vi "WireSelectionControl.vi"() -> ()   [LabVIEW 2020]
uses:
  resource/Framework/Providers/Open_GDS/SubVIs/GOOP_WireConfigurationType.ctl
  resource/Framework/Providers/Open_GDS/SubVIs/GOOP_WirePattern.ctl
  <vilib>/numeric/Random Number (Range) U64.vi
  <vilib>/numeric/sub_Random U32.vi
panel:
  out "Array":T1(array[cluster])
  out "Picture":picture
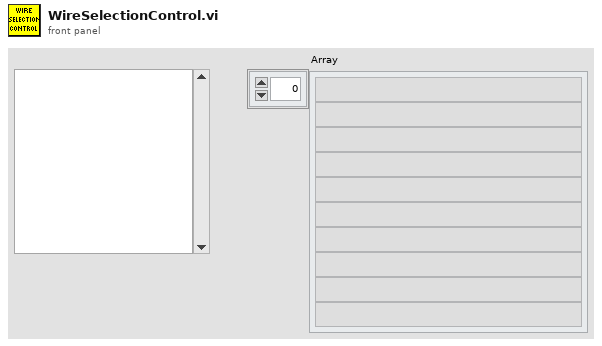
[diagram p1: front panel]
types:
  T1 = cluster{"Name":string, "Wire":picture, "Bg":picture}[]
  T2 = cluster{"left":i16, "top":i16, "right":i16, "bottom":i16}
  T3 = typedef "GOOP_WireConfigurationType.ctl" = cluster{"Edge thickness":i32, "Edge color":u32, "Center thickness":i32, "Center pattern":T4, "CenterColor1":u32, "CenterColor2":u32, "Tunnels and terminals colors":u32}
  T4 = typedef "GOOP_WirePattern.ctl" = enum16{"Solid", "Large dash", "Small dash"}
  T5 = cluster{"Width":i16, "Style":enum32{"Solid", "Dash", "Dot", "DashDot", "DashDotDot"}}
  T6 = cluster{"ImageEnd-Y":i32, i32, "rect":cluster{"left":i16, "top":i16, "right":i16, "bottom":i16}}
  T7 = cluster{string, "WirePictureOut":picture, "new picture":picture}
  T8 = typedef "LVMouseTypeDef.ctl" = cluster{"Mouse Position":cluster{"X":i32, "Y":i32}, "Mouse Modifiers":cluster{"Button Down":bool, "Shift Mod":bool, "Menu Mod":bool, "Option Mod":bool}}
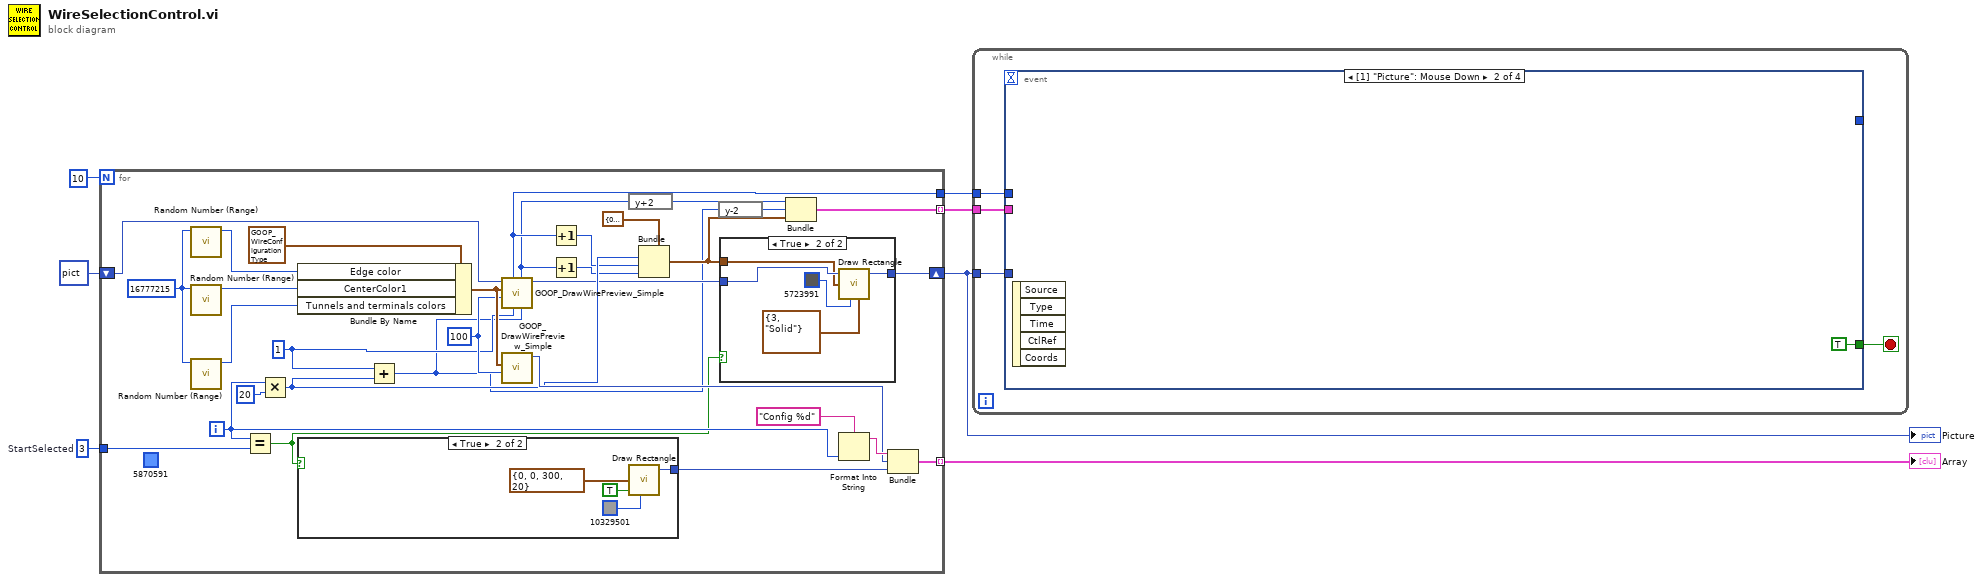
[diagram p0: block diagram]
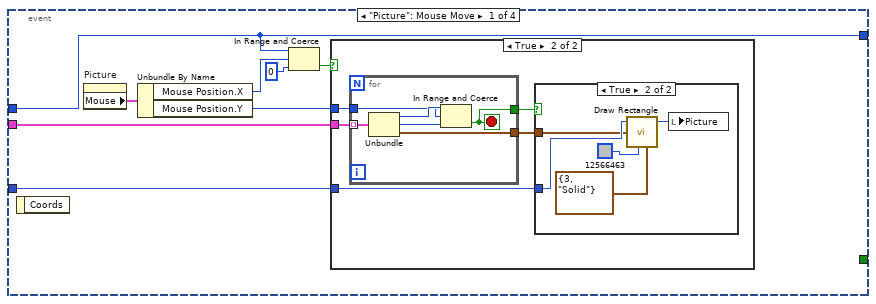
[diagram p2: hidden frame]
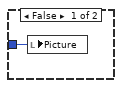
[diagram p3: hidden frame]
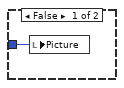
[diagram p4: hidden frame]
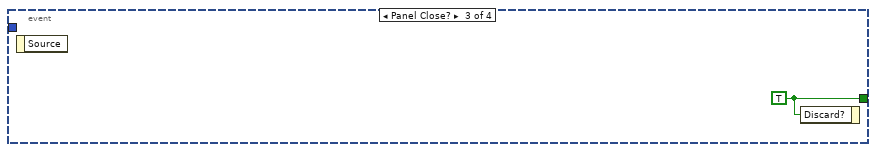
[diagram p5: hidden frame]
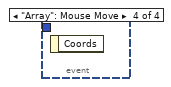
[diagram p6: hidden frame]
diagram:
  w5 = 3  # StartSelected
  n1 = for {
    N: 10 -> [_]
    shift-right: [w17] -> w3
    shift-left: picture data[5B] ("WirePictureOut") -> [w32]
    tunnel: [w28] -> w4 mode=indexing
    tunnel: w5 -> [w26]
    tunnel: [w20] -> w2 mode=indexing
    tunnel: [w19] -> w1
    i -> [w27]
    (unwired) u32 5870591 ("color(black)")
    w21 = i16 1 ("X-Offset")
    w35 = u64 16777215 ("upper bound (100)")
    w24 = i16 100 ("WireLength(X)")
    n2 = call-poly <vilib>:"Random Number (Range).vi"("upper bound (100)"=w35) -> ("number"=w36:u64)  [unwired: 10 in]
    n3 = call-poly <vilib>:"Random Number (Range).vi"("upper bound (100)"=w35) -> ("number"=w34:u64)  [unwired: 10 in]
    n4 = call-poly <vilib>:"Random Number (Range).vi"("upper bound (100)"=w35) -> ("number"=w33:u64)  [unwired: 10 in]
    n5 = Equal?(x=w27, y=w26) -> (x = y?=w12:bool)
    n6 = Multiply(x=w27, y=20) -> (x*y=w22:i32)
    n7 = Bundle By Name(cluster=T3 {"Edge thickness"=1, "Edge color"=6916708, "Center thickness"=1, "Center pattern"=enum."Solid", "CenterColor1"=8882055, "CenterColor2"=0, "Tunnels and terminals colors"=16711680} ("WireConfiguration"), "Edge color"=w36, "CenterColor1"=w34, "Tunnels and terminals colors"=w33) -> (w31:T3)
    n8 = case shown="True" w12 {
      tunnel: [_ w46] -> w25
      frame False {
      }
      frame True {
        n9 = call <vilib>:"Draw Rectangle.vi"("rect"=T2 {"left"=0, "top"=0, "right"=300, "bottom"=20}, "fill?(F)"=TRUE, "color(black)"=u32 10329501) -> ("new picture"=w46:picture)  [unwired: 6 in]
      }
    }
    n10 = Add(x=w21, y=w22) -> (x+y=w11:i32)
    n11 = call "GOOP_DrawWirePreview_Simple.vi"("Y-Offset"=w11, "X-Offset"=w21, "WireLength(100px)"=w24, "WireConfiguration"=w31, "PictureIn"=w32) -> ("WirePictureOut"=w18:picture, "ImageEnd-Y"=w10:i32, "ImageEnd-X"=w19:i32)  [unwired: 2 in, 2 out]
    n12 = call "GOOP_DrawWirePreview_Simple.vi"("WireLength(100px)"=w24, "WireConfiguration"=w31) -> ("WirePictureOut"=w29:picture)  [unwired: 5 in, 4 out]
    n13 = Increment(x=w19) -> (x+1=w13:i32)
    n14 = Increment(x=w10) -> (x+1=w14:i32)
    n15 = expression code="y+2"(w10) -> (w9:i32)
    n16 = Bundle(cluster=T2 {"left"=0, "top"=0, "right"=0, "bottom"=0} ("rect"), "top"=w22, "right"=w13, "bottom"=w14) -> (w16:T2)  [unwired: 1 in]
    n17 = expression code="y-2"(w11) -> (w8:i32)
    n18 = case shown="True" w12 {
      tunnel: w18 -> [w39 w44]
      tunnel: [w39 w43] -> w17
      tunnel: w16 -> [_ w42]
      frame False {
      }
      frame True {
        n19 = call <vilib>:"Draw Rectangle.vi"("picture"=w44, "rect"=w42, "color(black)"=u32 5723991, "pen"=T5 {"Width"=3, "Style"=enum."Solid"}) -> ("new picture"=w43:picture)  [unwired: 5 in]
      }
    }
    n20 = Bundle("ImageEnd-Y"=w9, w8, "rect"=w16) -> (w20:T6)  [unwired: 1 in]
    n21 = Format Into String(format string="Config %d", w27) -> (resulting string=w30:string)  [unwired: 2 in, 1 out]
    n22 = Bundle(w30, "WirePictureOut"=w29, "new picture"=w25) -> (w28:T7)  [unwired: 1 in]
  }
  "Picture" <- w3
  "Array" <- w4
  n23 = while {
    tunnel: w3 -> [w52]
    tunnel: w2 -> [w51]
    tunnel: w1 -> [w50]
    stop <- w49 stop-if-true
    n24 = event shown="[1] \"Picture\": Mouse Down" {
      selector: _ -> [_ _ _ _]
      dyn-events: _ -> [_ _ _ _]
      timeout: _ -> [_ _ _ _]
      tunnel: w52 -> [w53 _ _ _]
      tunnel: w51 -> [w59 _ _ _]
      tunnel: [w56 _ _ _] -> _
      tunnel: w50 -> [w56 _ _ _]
      tunnel: [_ TRUE ("Discard?") w80 _] -> w49
      event "Picture": Mouse Move {
        n25 = event-data() -> ()  [unwired: 1 in, 1 out]
        n26 = property on="Picture" class="Pict"() -> ("Mouse"=w60:T8)  [unwired: 2 in, 2 out]
        n27 = Unbundle By Name(w60) -> ("Mouse Position.X"=w58:i32, "Mouse Position.Y"=w54:i32)
        n28 = In Range and Coerce(upper limit=w56, x=w58, lower limit=0) -> (In Range?=w55:bool)  [unwired: 1 out]
        n29 = case shown="True" w55 {
          tunnel: w59 -> [_ w66]
          tunnel: w54 -> [_ w65]
          tunnel: w53 -> [w61 w63]
          frame False {
            n30 = local write "Picture"(w61) -> ()
          }
          frame True {
            n31 = for {
              tunnel: w66 -> [w78] mode=indexing
              tunnel: w65 -> [w75]
              tunnel: [w74] -> w64
              tunnel: [w73] -> w62
              stop <- w74 stop-if-true
              n32 = Unbundle(w78) -> ("ImageEnd-Y"=w76:i32, w77:i32, "rect"=w73:T2)
              n33 = In Range and Coerce(upper limit=w76, x=w75, lower limit=w77) -> (In Range?=w74:bool)  [unwired: 1 out]
            }
            n34 = case shown="True" w64 {
              tunnel: w63 -> [w67 w70]
              tunnel: w62 -> [_ w68]
              frame False {
                n35 = local write "Picture"(w67) -> ()
              }
              frame True {
                n36 = call <vilib>:"Draw Rectangle.vi"("picture"=w70, "rect"=w68, "color(black)"=u32 12566463, "pen"=T5 {"Width"=3, "Style"=enum."Solid"}) -> ("new picture"=w69:picture)  [unwired: 5 in]
                n37 = local write "Picture"(w69) -> ()
              }
            }
          }
        }
      }
      event "Picture": Mouse Down {
        n38 = event-data() -> ()  [unwired: 1 in, 5 out]
      }
      event Panel Close? {
        w80 = TRUE ("Discard?")
        n39 = event-data() -> ()  [unwired: 1 in, 1 out]
        n40 = event-data("Discard?"=w80) -> ()  [unwired: 1 in, 1 out]
      }
      event "Array": Mouse Move {
        n41 = event-data() -> ()  [unwired: 1 in, 1 out]
      }
    }
  }
